vi "Beam Scanning Cambridge V1.vi"() -> ()   [LabVIEW 2014]
uses:
  <vilib>/Platform/TimedLoop/XDataNode/timing_clust.ctl
  <vilib>/Platform/TimedLoop/XDataNode/nitl_modes.ctl
  <vilib>/Platform/TimedLoop/XDataNode/wakeup.ctl
  <vilib>/rvi/Emulation/niFpgaGetClockAttributes.vi
  <vilib>/rvi/Emulation/niFpgaSctlEmulationGetInTimedLoop.vi
  <vilib>/rvi/Emulation/niFpgaEmulationReportErrorSimple.vi
  <vilib>/rvi/Emulation/niFpgaProcessEmulError.vi
  <vilib>/rvi/Emulation/niFpgaCriticalErrorInLSC.vi
  <vilib>/rvi/Emulation/niFpgaEmulationIsFPGAContextNoSignature.vi
  <vilib>/rvi/errors/niFpgaSetErrorForExecOnDevCompSimple.vi
  <vilib>/rvi/eio/common/nirviEmuReportErrorAndStop.vi
  <vilib>/rvi/DataTransferAndStorage/Container/Common/niFpgaContainerGetUniqueNameForEmu.vi
  <vilib>/rvi/FIFO/Fifo_Resource/nirvififoEmulationSetSize.vi
  <vilib>/rvi/FIFO/Fifo_Resource/nirviFifoEmulationQueueMgr.vi
  <instcachedir>/0/nirviFifoEmulationQueueMgr_E5CAEC123FF24DC58D834DCA3CDAA9B5.lvgen/nirviFifoEmulationQueueMgr_E5CAEC123FF24DC58D834DCA3CDAA9B5_002.vi
  <vilib>/rvi/FIFO/Fifo_Resource/nirvififoEmulationDetermineInputValidOut.vi
  <vilib>/rvi/FIFO/Fifo_Resource/nirvififoEmulationCreateLock.vi
  <vilib>/rvi/FIFO/Fifo_Resource/nirvififoEmulationObtainLock.vi
  <vilib>/rvi/FIFO/Fifo_Resource/nirvififoEmulationReleaseLock.vi
  <vilib>/rvi/occurrence/nirviWaitOnOccurrenceBase.vi
  <vilib>/rvi/errors/nirviReportUnexpectedCaseInternalError.vi
  <vilib>/rvi/errors/nirviReportUnexpectedCaseInternalError (U32).vi
  <instcachedir>/0/nirviFifoEmulationQueueMgr_E5CAEC123FF24DC58D834DCA3CDAA9B5.lvgen/nirviFifoEmulationQueueMgr_E5CAEC123FF24DC58D834DCA3CDAA9B5_001.vi
  <vilib>/Utility/error.llb/Clear Errors.vi
  <vilib>/rvi/Memory/Memory_Emulation/nirvimemoryFastEmulation.vi
  <vilib>/rvi/Memory/Memory_Emulation/nirvimemoryEmulation.vi
  <vilib>/rvi/eio/common/nirviEmuTemplateMethod_errors.vi
  <instcachedir>/0/nirviFifoEmulationQueueMgr_E5CAEC123FF24DC58D834DCA3CDAA9B5.lvgen/nirviFifoEmulationQueueMgr_E5CAEC123FF24DC58D834DCA3CDAA9B5_000.vi
  <vilib>/rvi/interface/RandomDataEmulation/niFpgaRandomDataHandleErrors.vi
  <vilib>/rvi/DataTransferAndStorage/Container/XNode/niFpgaContainer.xnode
  <vilib>/rvi/FIFO/Fifo_Resource/nirvififoEmulationWrite.vi
  <vilib>/Platform/TimedLoop/XDataNode/XDataNode.xnode
  <vilib>/rvi/FIFO/Fifo_Resource/nirvififoEmulationRead.vi
  <vilib>/eio/EIONode/EIONode.xnode
  <vilib>/rvi/interface/RandomDataEmulation/nirviRandomDataFpgaReadWriteTemplate.vi
  <vilib>/Platform/TimedLoop/XDataNode/XDNodeRunTimeDep.lvlib
panel:
  in  "Stop Acquisition":bool
  in  "Accums Per Line":u16[](array[numeric])=[0, 0, 0, 0]
  in  "Sequences":u8=4
  in  "Line Trigger":bool
  in  "Dead Lines":u16
  in  "Lines Per Image":u16
  in  "Trigger Delay (Ticks)":u16=1125
  in  "FPGA Samples":i32=4000
  out "Ready For Write":bool
  in  "BinEdge":bool
  in  "PreBinnedValue":u32
  # "V3 - Updated AO and switched to dead lines, not dead time.\nV4 - Attempting to use logistics function for AO.\nV5 - Switch from DIO2 as loop trigger to FIFO.\n20120919 - Deleting analog out as this will be done with the analog card.\n20120928 - Adding in analog control for the Y galvo.\n20121001 - Removing Y galvo analog control. Adding analog out for x-axis resmirror amplitude setting.\n20121004 - Adding laser power control for live preview mode.\n20121205 - V10 Starting the multi channel upgrade\n20130116 - V11 Turn off lasers when the program starts\n20130117 - V12 Attemp to add beam blanking and line switching\n20130118 - V13 - Blanking and switching work, added in line accums for the lasers on\n20130118 - V14 - Add varrying line accums\n20130509 - V16 - Took out the res mirror amplitude control and added in a blanking on/off option\n20130531 - V17 Fixing laser on accums trigger problem"
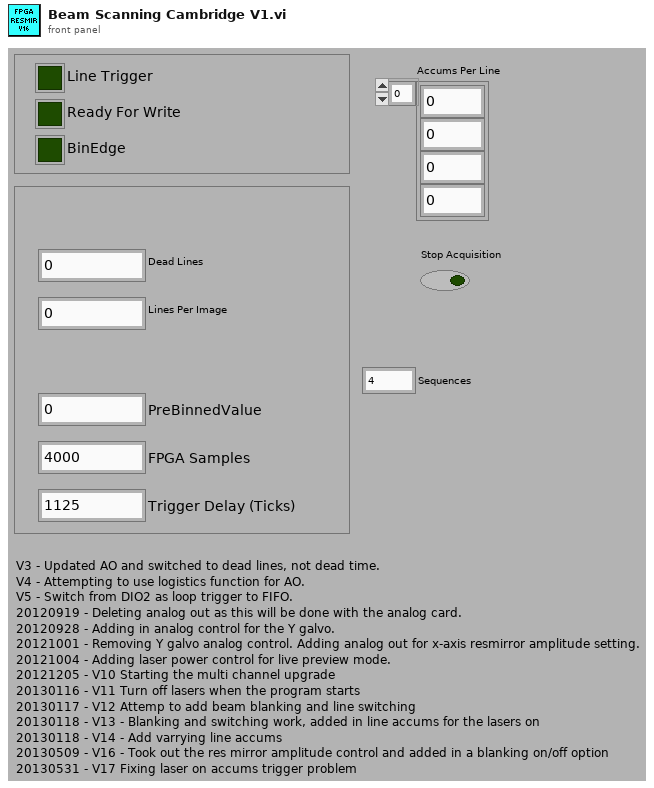
[diagram p1: front panel]
types:
  T1 = typedef "XDNodeRunTimeDep.lvlib/timing_clust.ctl" = cluster{"Expected End [f-1]":u64, "Actual End [f-1]":u64, "Finished Late? [f-1]":bool, "Expected End [i-1]":u64, "Actual End [i-1]":u64, "Finished Late? [i-1]":bool, "Expected Start [i]":u64, "Actual Start [i]":u64, "Expected Start [f]":u64, "Actual Start [f]":u64, "Source Name":string, "Structure Name":string, "Period":i64, "Deadline":i64, "Offset":i64, "Start":i64, "Priority":i32, "Timeout":i32, "Mode":T2, "Wakeup Reason":T3, "Error":errorcluster, "Source Type":string, "Secondary Source Type":string, "Global End Time":u64, "Global Start Time":u64, "Frame Duration":u64, "Iteration Duration":u64, "Assigned CPU":i32, "I/O Scan Engine Mode":u32}
  T2 = typedef "XDNodeRunTimeDep.lvlib/nitl_modes.ctl" = enum32{"No Change", "Process missed periods, maintain original phase", "Discard missed periods, maintain original phase", "Process missed periods, ignore original phase", "Discard missed periods, ignore original phase"}
  T3 = typedef "XDNodeRunTimeDep.lvlib/wakeup.ctl" = enum32{"Normal", "Aborted", "Asynchronous wakeup", "Timing source error", "Timed loop error", "Timeout"}
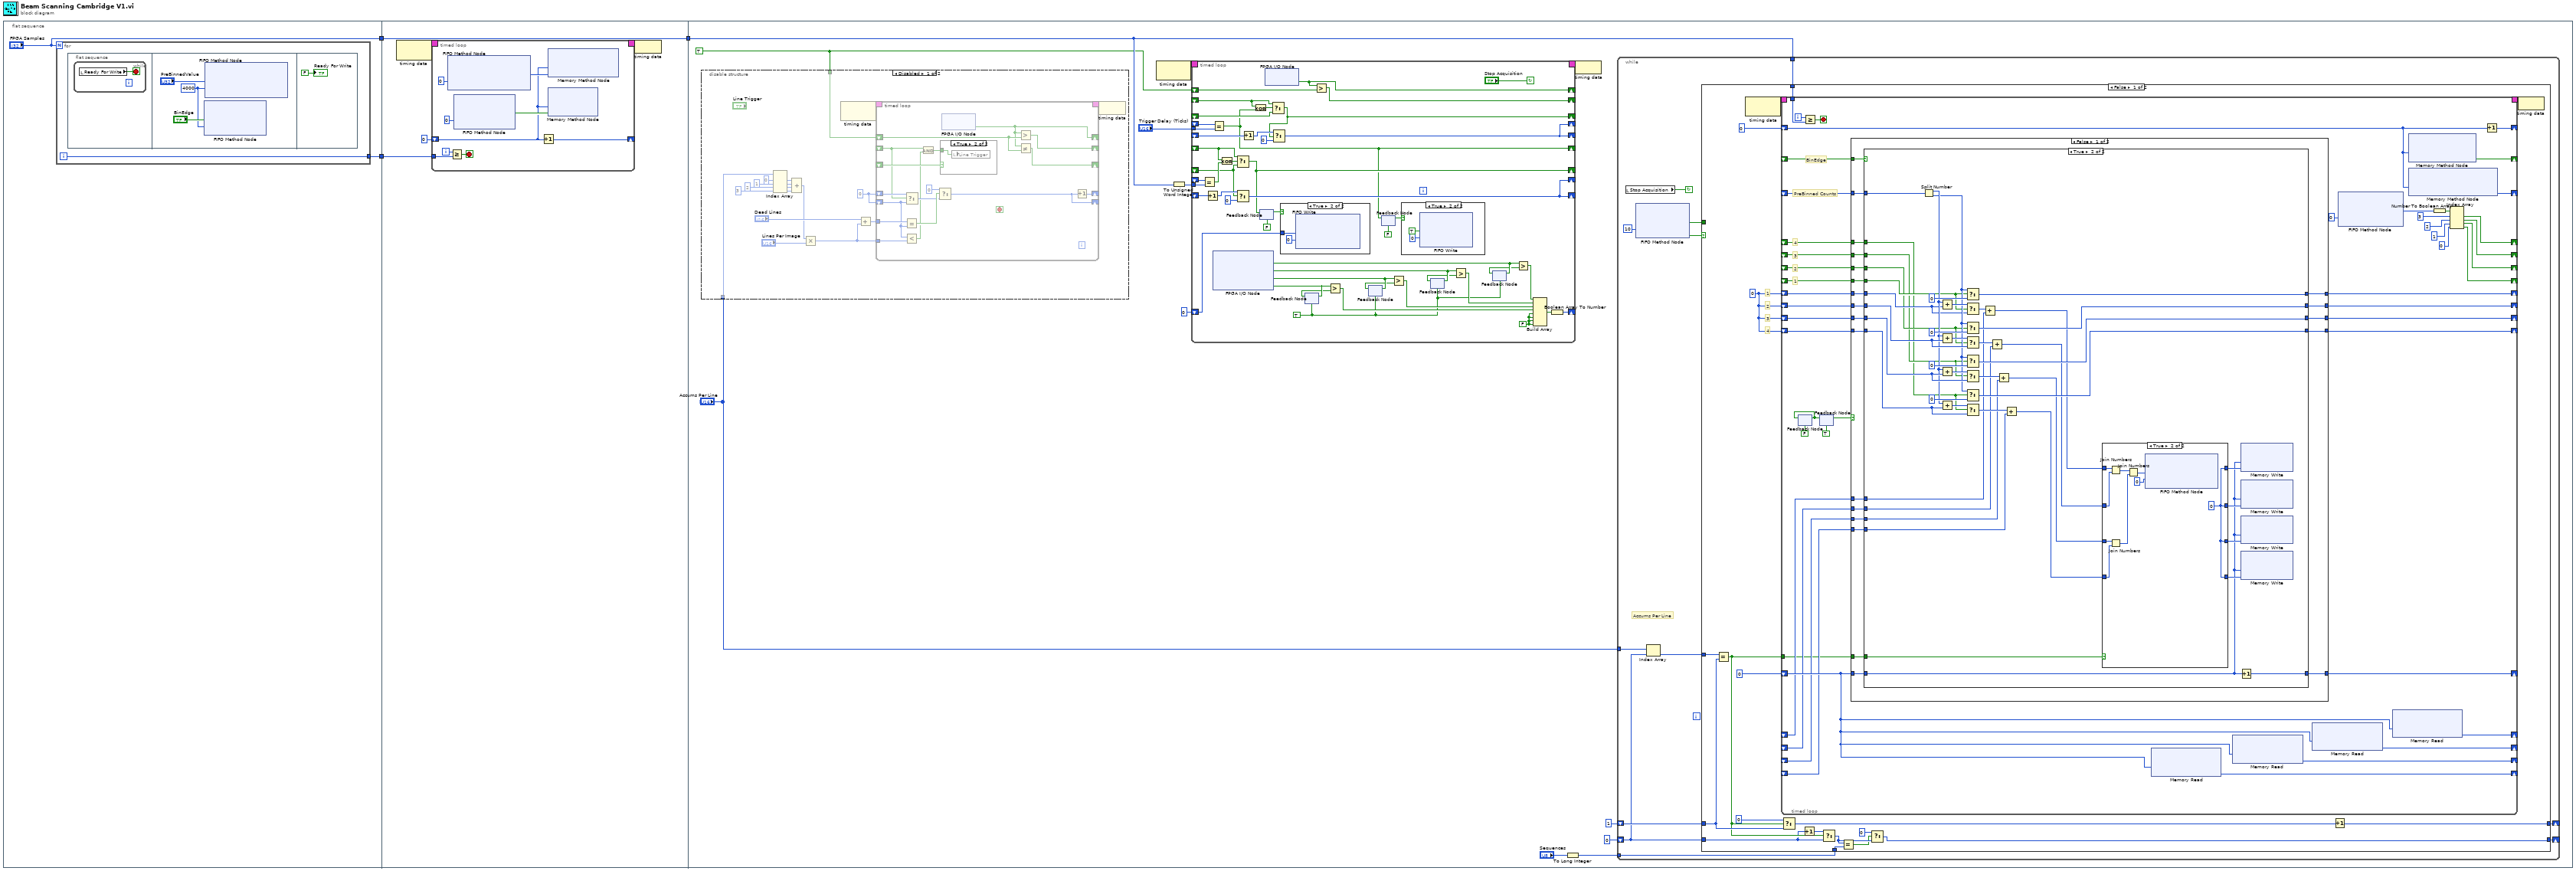
[diagram p0: block diagram]
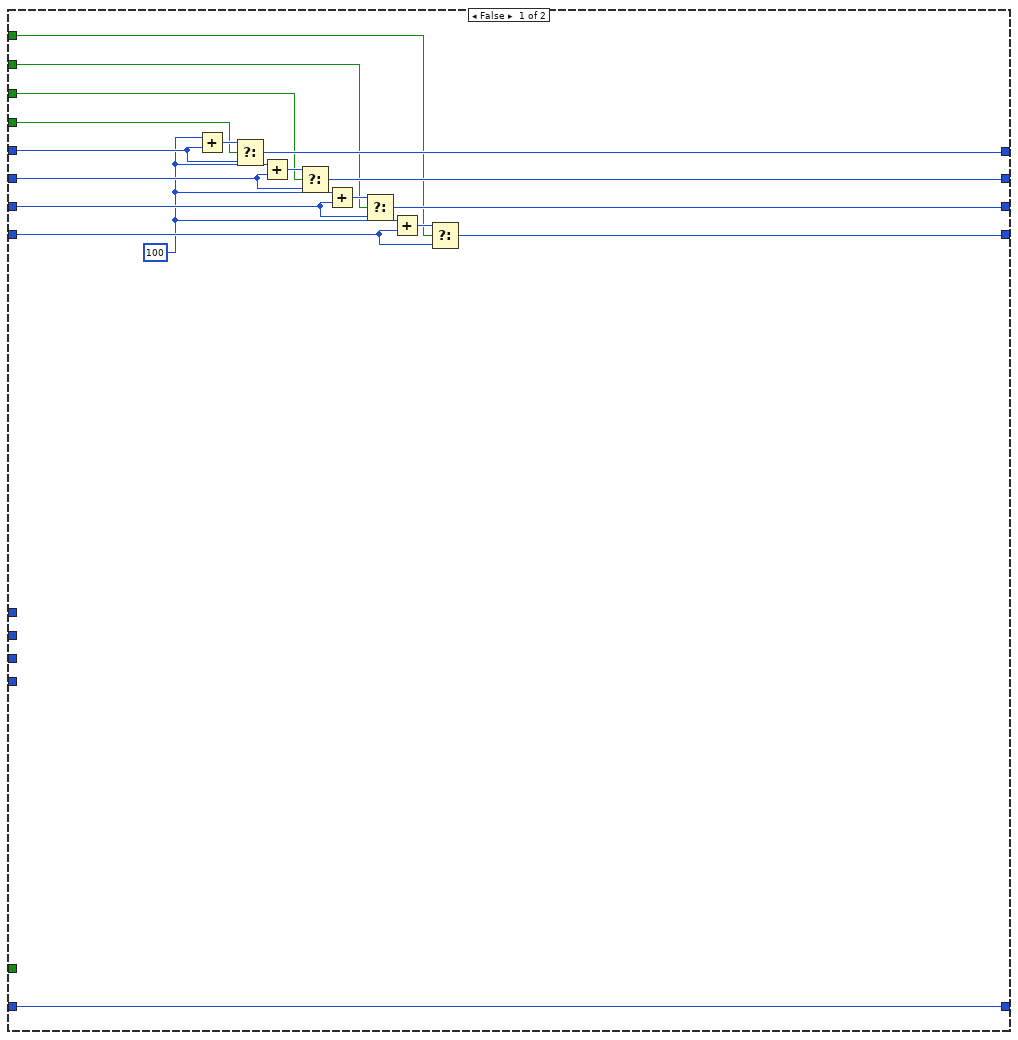
[diagram p6: hidden frame]
diagram:
  n1 = flat-sequence {
    tunnel: ["FPGA Samples"] -> w3
    tunnel: [w4] -> w1
    tunnel: w3 -> [w13]
    tunnel: [w13] -> w2
    tunnel: w1 -> [w12]
    tunnel: w2 -> [w40]
    frame #0 {
      n2 = for {
        N: "FPGA Samples" -> [_]
        tunnel: [w6] -> w4
        i -> [w6]
        n3 = flat-sequence {
          frame #0 {
            n4 = while {
              stop <- w7 stop-if-true
              n5 = local read "Ready For Write"() -> (w7:bool)
            }
          }
          frame #1 {
            w8 = 4000 ("Timeout")
            n6 = xnode ("FIFO Method Node")("Element"="BinEdge", "Timeout"=w8) -> ()  [unwired: 1 in, 2 out]
            n7 = xnode ("FIFO Method Node")("Element"="PreBinnedValue", "Timeout"=w8) -> ()  [unwired: 1 in, 2 out]
          }
          frame #2 {
            "Ready For Write" <- FALSE ("Ready For Write")
          }
        }
      }
    }
    frame #1 {
      n8 = node-c288() -> (w16:T1)  [unwired: 1 in]
      n9 = timed-loop {
        timing: w16 -> [_]
        timing-out: [_] -> w15
        shift-right: [w20] -> _
        shift-left: u32 0 ("Address") -> [w21]
        tunnel: w12 -> [w17]
        i -> [w19]
        stop <- w18 stop-if-true
        n10 = xnode ("FIFO Method Node")("Timeout"=0) -> ("Element"=w23:u32)  [unwired: 1 in, 2 out]
        n11 = Greater Or Equal?(x=w19, y=w17) -> (x >= y?=w18:bool)
        n12 = xnode ("FIFO Method Node")("Timeout"=0) -> ("Element"=w22:bool)  [unwired: 1 in, 2 out]
        n13 = Increment(x=w21) -> (x+1=w20:u32)
        n14 = xnode ("Memory Method Node")("Address"=w21, "Data"=w23) -> ()  [unwired: 1 in, 1 out]
        n15 = xnode ("Memory Method Node")("Address"=w21, "Data"=w22) -> ()  [unwired: 1 in, 1 out]
      }
      n16 = node-c288(w15) -> ()
    }
    frame #2 {
      w30 = TRUE
      n17 = disable-structure shown="Disabled" {
        disable-tunnel: "Accums Per Line" -> [w45 _]
        disable-tunnel: w30 -> [w42 _]
        frame Disabled {
          w44 = u16 0
          n18 = Index Array(array=w45, index #1=0 ("index"), index #2=1 ("index"), index #3=2 ("index"), index #4=3 ("index")) -> (element #1=w51:u16, element #2=w52:u16, element #3=w53:u16, element #4=w54:u16)
          n19 = Compound Arithmetic op=ADD(w51, w52, w53, w54) -> (w46:u16)
          n20 = Multiply(x=w46, y="Lines Per Image") -> (x*y=w55:u16)
          n21 = node-c288() -> (w59:T1)  [unwired: 1 in]
          n22 = Add(x="Dead Lines", y=w55) -> (x+y=w43:u16)
          n23 = timed-loop {
            shift-right: [w67] -> _
            shift-left: w42 -> [w76]
            shift-right: [w63] -> _
            shift-left: _ -> [w60]
            shift-right: [w74] -> _
            shift-left: _ -> [w64]
            shift-right: [w73] -> _
            shift-left: w44 -> [w75]
            shift-right: [w66] -> _
            shift-left: w44 -> [w62]
            tunnel: w55 -> [w70]
            tunnel: w43 -> [w71]
            timing: w59 -> [_]
            timing-out: [_] -> w58
            stop <- _ stop-if-true
            n24 = Select(t=w75, s=w60, f=w62) -> (s? t:f=w68:u16)
            n25 = Equal?(x=w71, y=w62) -> (x = y?=w69:bool)
            n26 = Less?(x=w62, y=w70) -> (x < y?=w61:bool)
            n27 = And(x=w60, y=w61) -> (x .and. y?=w65:bool)
            n28 = Select(t=u16 0, s=w69, f=w68) -> (s? t:f=w66:u16)
            n29 = case shown="True" w64 {
              tunnel: w65 -> [_ w77]
              frame False {
              }
              frame True {
                n30 = local write "Line Trigger"(w77) -> ()
              }
            }
            n31 = xnode "FPGA I/O Node"() -> ("RTSI1"=w67:bool)  [unwired: 1 in, 1 out]
            n32 = Greater?(x=w67, y=w76) -> (0:w63:bool)
            n33 = Not Equal?(x=w67, y=w76) -> (x != y?=w74:bool)
            n34 = Increment(x=w66) -> (x+1=w73:u16)
          }
          n35 = node-c288(w58) -> ()
        }
        frame Enabled {
        }
      }
      n36 = node-c288() -> (w39:T1)  [unwired: 1 in]
      n37 = To Unsigned Word Integer(number=w40) -> (unsigned 16bit integer=w36:u16)
      n38 = timed-loop {
        timing: w39 -> [_]
        timing-out: [_] -> w38
        shift-right: [w113] -> _
        shift-left: _ -> [w108]
        shift-right: [w109] -> _
        shift-left: _ -> [w124]
        shift-right: [w123] -> _
        shift-left: _ -> [w126]
        shift-right: [w123] -> _
        shift-left: _ -> [w122]
        shift-right: [w86] -> _
        shift-left: _ -> [w121]
        shift-right: [w89] -> _
        shift-left: _ -> [w110]
        shift-right: [w117] -> _
        shift-left: _ -> [w116]
        shift-right: [w117] -> _
        shift-left: _ -> [w118]
        shift-right: [w83] -> _
        shift-left: w30 -> [w114]
        tunnel: w36 -> [w112]
        tunnel: "Trigger Delay (Ticks)" -> [w111]
        shift-right: [w92] -> _
        shift-left: u8 0 -> [w91]
        stop <- "Stop Acquisition" continue-if-true
        w84 = FALSE ("element")
        w94 = TRUE
        n39 = Equal?(x=w116, y=w112) -> (x = y?=w115:bool)
        n40 = Increment(x=w118) -> (x+1=w120:u16)
        n41 = Equal?(x=w122, y=w111) -> (x = y?=w86:bool)
        n42 = xnode "FPGA I/O Node"() -> ("Connector1/DIO0"=w100:bool, "Connector1/DIO1"=w102:bool, "Connector1/DIO2"=w104:bool, "Connector1/DIO3"=w106:bool)  [unwired: 4 in, 4 out]
        n43 = Exclusive Or(1:w115, 2:w121) -> (0:w107:bool)
        n44 = Select(t=w121, s=w107, f=w110) -> (s? t:f=w89:bool)
        n45 = Select(t=w120, s=w110, f=u16 0) -> (s? t:f=w117:u16)
        n46 = Increment(x=w126) -> (x+1=w125:u16)
        n47 = Exclusive Or(1:w86, 2:w108) -> (0:w128:bool)
        n48 = feedback-in #1(w89) -> ()
        n49 = feedback #1(FALSE) -> (w88:bool)
        n50 = xnode "FPGA I/O Node"() -> ("RTSI1"=w83:bool)  [unwired: 1 in, 1 out]
        n51 = Select(t=w108, s=w128, f=w124) -> (s? t:f=w109:bool)
        n52 = Select(t=w125, s=w109, f=u16 0) -> (s? t:f=w123:u16)
        n53 = case shown="True" w88 {
          tunnel: w91 -> [_ w131]
          frame False {
          }
          frame True {
            n54 = xnode ("FIFO Write")("Element"=w131, "Timeout"=0) -> ()  [unwired: 1 in, 2 out]
          }
        }
        n55 = feedback #2(w94) -> (w105:bool)
        n56 = feedback-in #2(w106) -> ()
        n57 = Greater?(x=w83, y=w114) -> (0:w113:bool)
        n58 = Greater?(x=w106, y=w105) -> (0:w95:bool)
        n59 = feedback #3(w94) -> (w103:bool)
        n60 = feedback-in #3(w104) -> ()
        n61 = feedback-in #4(w86) -> ()
        n62 = feedback #4(FALSE) -> (w85:bool)
        n63 = Greater?(x=w104, y=w103) -> (0:w96:bool)
        n64 = case shown="True" w85 {
          frame False {
          }
          frame True {
            n65 = xnode ("FIFO Write")("Element"=TRUE, "Timeout"=0) -> ()  [unwired: 1 in, 2 out]
          }
        }
        n66 = feedback #5(w94) -> (w101:bool)
        n67 = feedback-in #5(w102) -> ()
        n68 = Greater?(x=w102, y=w101) -> (0:w97:bool)
        n69 = feedback #6(w94) -> (w99:bool)
        n70 = feedback-in #6(w100) -> ()
        n71 = Greater?(x=w100, y=w99) -> (0:w98:bool)
        n72 = Build Array(w98, w97, w96, w95, w84, w84, w84, w84) -> (w93:bool[])
        n73 = Boolean Array To Number(Boolean array=w93) -> (number=w92:u8)
      }
      n74 = To Long Integer(number="Sequences") -> (32bit integer=w31:i32)
      n75 = node-c288(w38) -> ()
      n76 = while {
        tunnel: w40 -> [w148]
        shift-right: [w146] -> _
        shift-left: u16 1 -> [w147]
        tunnel: "Accums Per Line" -> [w142]
        shift-right: [w139] -> _
        shift-left: 0 -> [w140]
        tunnel: w31 -> [w138]
        stop <- w137 continue-if-true
        # "Accums Per Line"
        n77 = local read "Stop Acquisition"() -> (w137:bool)
        n78 = xnode ("FIFO Method Node")("Timeout"=10) -> ("Element"=w143:bool, "Timed Out?"=w144:bool)  [unwired: 1 in, 1 out]
        n79 = Index Array(array=w142, index=w140) -> (element=w141:u16)
        n80 = case shown="False" w144 {
          tunnel: w148 -> [w167 _]
          tunnel: w147 -> [w165 w319]
          tunnel: [w166 w319] -> w146
          tunnel: w143 -> [_ _]
          tunnel: w141 -> [w157 _]
          tunnel: w140 -> [w154 w318]
          tunnel: [w152 w318] -> w139
          tunnel: w138 -> [w150 _]
          frame False {
            w159 = u16 0
            # "4"
            # "3"
            # "2"
            # "1"
            n81 = Equal?(x=w157, y=w165) -> (x = y?=w156:bool)
            n82 = node-c288() -> (w162:T1)  [unwired: 1 in]
            n83 = timed-loop {
              timing: w162 -> [_]
              timing-out: [_] -> w161
              tunnel: w167 -> [w211]
              shift-right: [w171] -> _
              shift-left: _ -> [w198]
              shift-right: [w170] -> _
              shift-left: _ -> [w197]
              shift-right: [w169] -> _
              shift-left: _ -> [w196]
              shift-right: [w168] -> _
              shift-left: _ -> [w195]
              shift-right: [w208] -> _
              shift-left: _ -> [w184]
              shift-right: [w207] -> _
              shift-left: _ -> [w183]
              shift-right: [w206] -> _
              shift-left: _ -> [w182]
              shift-right: [w205] -> _
              shift-left: _ -> [w181]
              shift-right: [w204] -> _
              shift-left: u32 0 ("Address") -> [w203]
              shift-right: [w191] -> _
              shift-left: w159 -> [w202]
              shift-right: [w192] -> _
              shift-left: w159 -> [w201]
              shift-right: [w193] -> _
              shift-left: w159 -> [w200]
              shift-right: [w194] -> _
              shift-left: w159 -> [w199]
              shift-right: [w190] -> _
              shift-left: _ -> [w188]
              shift-right: [w189] -> _
              shift-left: _ -> [w186]
              shift-right: [w185] -> _
              shift-left: u32 0 ("Address") -> [w187]
              tunnel: w156 -> [w180]
              i -> [w213]
              stop <- w212 stop-if-true
              # "PreBinned Counts"
              # "BinEdge"
              # "4"
              # "3"
              # "2"
              # "1"
              n84 = feedback #7(FALSE) -> (w179:bool)
              n85 = feedback-in #7(w179) -> ()
              n86 = Greater Or Equal?(x=w213, y=w211) -> (x >= y?=w212:bool)
              n87 = feedback #8(TRUE) -> (w177:bool)
              n88 = feedback-in #8(w179) -> ()
              n89 = case shown="False" w177 {
                tunnel: [w235 w309] -> w204
                tunnel: w203 -> [w234 w309]
                tunnel: w202 -> [w233 w313]
                tunnel: w201 -> [w232 w312]
                tunnel: w200 -> [w231 w311]
                tunnel: w199 -> [w230 w310]
                tunnel: w198 -> [w229 _]
                tunnel: w197 -> [w228 _]
                tunnel: w196 -> [w227 _]
                tunnel: w195 -> [w226 _]
                tunnel: [w225 w310] -> w194
                tunnel: [w224 w311] -> w193
                tunnel: [w223 w312] -> w192
                tunnel: [w222 w313] -> w191
                tunnel: w188 -> [w221 _]
                tunnel: w186 -> [w220 _]
                tunnel: w184 -> [w219 _]
                tunnel: w183 -> [w218 _]
                tunnel: w182 -> [w217 _]
                tunnel: w181 -> [w216 _]
                tunnel: w180 -> [w215 _]
                frame False {
                  n90 = case shown="True" w221 {
                    tunnel: w234 -> [w253 w254]
                    tunnel: [w253 w295] -> w235
                    tunnel: w233 -> [w247 w272]
                    tunnel: w232 -> [w250 w280]
                    tunnel: w231 -> [w249 w279]
                    tunnel: w230 -> [w248 w278]
                    tunnel: w229 -> [w236 w255]
                    tunnel: w228 -> [w237 w256]
                    tunnel: w227 -> [w238 w257]
                    tunnel: w226 -> [w239 w258]
                    tunnel: [w244 w273] -> w225
                    tunnel: [w243 w274] -> w224
                    tunnel: [w242 w275] -> w223
                    tunnel: [w241 w292] -> w222
                    tunnel: w220 -> [_ w294]
                    tunnel: w219 -> [_ w271]
                    tunnel: w218 -> [_ w270]
                    tunnel: w217 -> [_ w269]
                    tunnel: w216 -> [_ w268]
                    tunnel: w215 -> [_ w259]
                    frame False {
                      w240 = u16 100
                      n91 = Add(x=w240, y=w247) -> (x+y=w252:u16)
                      n92 = Select(t=w252, s=w239, f=w247) -> (s? t:f=w241:u16)
                      n93 = Add(x=w240, y=w250) -> (x+y=w251:u16)
                      n94 = Select(t=w251, s=w238, f=w250) -> (s? t:f=w242:u16)
                      n95 = Add(x=w240, y=w249) -> (x+y=w246:u16)
                      n96 = Select(t=w246, s=w237, f=w249) -> (s? t:f=w243:u16)
                      n97 = Add(x=w240, y=w248) -> (x+y=w245:u16)
                      n98 = Select(t=w245, s=w236, f=w248) -> (s? t:f=w244:u16)
                    }
                    frame True {
                      n99 = Split Number(x=w294) -> (hi(x)=w277:u16, lo(x)=w276:u16)
                      n100 = Add(x=w277, y=w272) -> (x+y=w291:u16)
                      n101 = Add(x=w277, y=w280) -> (x+y=w288:u16)
                      n102 = Add(x=w277, y=w279) -> (x+y=w285:u16)
                      n103 = Add(x=w277, y=w278) -> (x+y=w282:u16)
                      n104 = Select(t=w276, s=w258, f=u16 0) -> (s? t:f=w292:u16)
                      n105 = Select(t=w291, s=w258, f=w272) -> (s? t:f=w290:u16)
                      n106 = Select(t=w276, s=w257, f=u16 0) -> (s? t:f=w275:u16)
                      n107 = Select(t=w288, s=w257, f=w280) -> (s? t:f=w289:u16)
                      n108 = Select(t=w276, s=w256, f=u16 0) -> (s? t:f=w274:u16)
                      n109 = Select(t=w285, s=w256, f=w279) -> (s? t:f=w284:u16)
                      n110 = Select(t=w276, s=w255, f=u16 0) -> (s? t:f=w273:u16)
                      n111 = Select(t=w282, s=w255, f=w278) -> (s? t:f=w283:u16)
                      n112 = Add(x=w290, y=w271) -> (x+y=w260:u16)
                      n113 = Add(x=w289, y=w270) -> (x+y=w261:u16)
                      n114 = Add(x=w284, y=w269) -> (x+y=w262:u16)
                      n115 = Add(x=w283, y=w268) -> (x+y=w263:u16)
                      n116 = case shown="True" w259 {
                        tunnel: [w296 w308] -> w267
                        tunnel: [w297 w308] -> w266
                        tunnel: [w298 w308] -> w265
                        tunnel: [w299 w308] -> w264
                        tunnel: w263 -> [w299 w304]
                        tunnel: w262 -> [w298 w306]
                        tunnel: w261 -> [w297 w305]
                        tunnel: w260 -> [w296 w307]
                        frame False {
                        }
                        frame True {
                          w308 = u16 0 ("Data")
                          n117 = Join Numbers(hi=w307, lo=w305) -> ((hi.lo)=w302:u32)
                          n118 = Join Numbers(hi=w306, lo=w304) -> ((hi.lo)=w300:u32)
                          n119 = Join Numbers(hi=w302, lo=w300) -> ((hi.lo)=w301:u64)
                          n120 = xnode ("FIFO Method Node")("Element"=w301, "Timeout"=0) -> ()  [unwired: 1 in, 2 out]
                        }
                      }
                      n121 = Increment(x=w254) -> (x+1=w295:u32)
                      n122 = xnode ("Memory Write")("Address"=w254, "Data"=w267) -> ()  [unwired: 1 in, 1 out]
                      n123 = xnode ("Memory Write")("Address"=w254, "Data"=w266) -> ()  [unwired: 1 in, 1 out]
                      n124 = xnode ("Memory Write")("Address"=w254, "Data"=w265) -> ()  [unwired: 1 in, 1 out]
                      n125 = xnode ("Memory Write")("Address"=w254, "Data"=w264) -> ()  [unwired: 1 in, 1 out]
                    }
                  }
                }
                frame True {
                }
              }
              n126 = xnode ("Memory Read")("Address"=w203) -> ("Data"=w205:u16)  [unwired: 1 in, 1 out]
              n127 = xnode ("Memory Read")("Address"=w203) -> ("Data"=w206:u16)  [unwired: 1 in, 1 out]
              n128 = xnode ("Memory Read")("Address"=w203) -> ("Data"=w207:u16)  [unwired: 1 in, 1 out]
              n129 = xnode ("FIFO Method Node")("Timeout"=0) -> ("Element"=w210:u8)  [unwired: 1 in, 2 out]
              n130 = xnode ("Memory Read")("Address"=w203) -> ("Data"=w208:u16)  [unwired: 1 in, 1 out]
              n131 = xnode ("Memory Method Node")("Address"=w187) -> ("Data"=w190:bool)  [unwired: 1 in, 1 out]
              n132 = xnode ("Memory Method Node")("Address"=w187) -> ("Data"=w189:u32)  [unwired: 1 in, 1 out]
              n133 = Number To Boolean Array(number=w210) -> (Boolean array=w209:bool[])
              n134 = Index Array(array=w209, index #1=3 ("index"), index #2=2 ("index"), index #3=1 ("index"), index #4=0 ("index")) -> (element #1=w171:bool, element #2=w170:bool, element #3=w169:bool, element #4=w168:bool)
              n135 = Increment(x=w187) -> (x+1=w185:u32)
            }
            n136 = Select(t=u16 0, s=w156, f=w165) -> (s? t:f=w164:u16)
            n137 = Increment(x=w154) -> (x+1=w155:i32)
            n138 = Select(t=w155, s=w156, f=w154) -> (s? t:f=w151:i32)
            n139 = Equal?(x=w151, y=w150) -> (x = y?=w149:bool)
            n140 = Select(t=0, s=w149, f=w151) -> (s? t:f=w152:i32)
            n141 = Increment(x=w164) -> (x+1=w166:u16)
            n142 = node-c288(w161) -> ()
          }
          frame True {
          }
        }
      }
    }
  }
